vi "Read Results.vi"(8 "error in (no error)":errorcluster, 11 "Project Builder in":refnum<class "Project Builder.lvclass">) -> (0 "error out":errorcluster, 2 "Results":T1[](array[typedef]), 3 "Project Builder out":refnum<class "Project Builder.lvclass">)   [LabVIEW 2020, in "ProjectBuilder.lvlib" / "Project Builder.lvclass"]
uses:
  Project Builder.lvclass
  Data/Report Data/Report Data.lvclass
  Action/Project Action/Project Action.lvclass
  Ctl/Ctl_Build Steps.ctl
  ProjectBuilder.lvlib
  Ctl/Ctl_Action Result.ctl
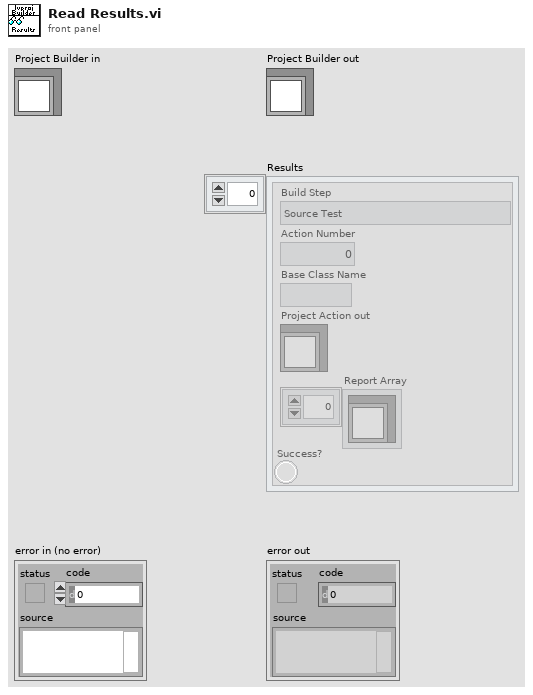
[diagram p1: front panel]
types:
  T1 = typedef "ProjectBuilder.lvlib/Ctl_Action Result.ctl" = cluster{"Build Step":T2, "Action Number":i32, "Base Class Name":string, "Project Action out":refnum<class "Project Action.lvclass">, "Report Array":refnum<class "Report Data.lvclass">[], "Success?":bool}
  T2 = typedef "ProjectBuilder.lvlib/Ctl_Build Steps.ctl" = enum16{"Source Test", "Build", "Post-Build Test", "Deploy", "Report"}
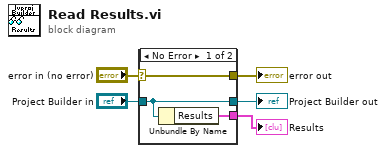
[diagram p0: block diagram]
diagram:
  n1 = case shown="No Error" "error in (no error)" {
    selector: "error in (no error)" -> [w8 w9]
    tunnel: [w8 w9] -> w4
    tunnel: [w7 w10] -> w2
    tunnel: "Project Builder in" -> [w7 w10]
    tunnel: [w6 _] -> w1
    frame No Error {
      n2 = Unbundle By Name(w7) -> ("Results"=w6:T1[])
    }
    frame Error {
    }
  }
  "error out" <- w4
  "Project Builder out" <- w2
  "Results" <- w1
